vi "FOCUS_V42_H37.vi"(9 "X-pixels":sgl=256.0 min=2 step=2, 11 "Run":bool) -> (0 "Retrace pixels":sgl=32.0 min=2 step=2, 10 "Pixel Clock (Hz)":sgl=170000.0)   [LabVIEW 2010]
doc: "This Labview program is the user interface for a 2 photon imaging system. The acquisition and control hardware consists of 3 commercial boards from National Instruments. A PCI-6110E 4 channel 5MS/S 12 bit simultaneous-sampling analog input board is used for acquiring data. Two PCI-6711 analog output boards are used to generate the X and Y waveforms which drive the scanning mirrors. A number of custom VIs are used in addition to the standard VIs available with the base Labview development system and the Labview Vision module.\n\nDeveloped for the Kleinfeld Lab in the Physics Dept. at UCSD.\nRelease 1. May 2003."
uses:
  <vilib>/DAQmx/write.llb/DAQmx Write.vi
  <vilib>/DAQmx/create/channels.llb/DAQmx Create Virtual Channel.vi
  <vilib>/DAQmx/read.llb/DAQmx Read.vi
  <vilib>/DAQmx/configure/trigger.llb/DAQmx Trigger.vi
  <vilib>/DAQmx/configure/timing.llb/DAQmx Timing.vi
  <vilib>/Analysis/baseanly.llb/Real A x B.vi
  <vilib>/Analysis/NI_AALBase.lvlib
  <vilib>/Utility/inputDevices.llb/Close Input Device.vi
  FOCUS_V4.llb/GlobelFSCOPE.vi
  Program Files/National Instruments/LabVIEW 2010/resource/objmgr/daqmx.rc
  <vilib>/Analysis/1siggen.llb/Ramp Pattern by Samples.vi
panel:
  in  "Case Constant\n(See Context Help)":bool
  in  "Notebook Window":string="Date:\nType of experiment:\nStaining: "
  in  "Modes":T1(tab)=enum."Parameters"
  in  "Channel selector":u8(ring) items=["Green and Red", "Green and Blue", "Blue and Red", "Green and Red (and Blue)", "Green and Blue (and Red)", "Blue and Red (and Green)"]
  in  "Linescan mode":bool caption="Vertical\n\n\nHorizontal"
  in  "Focus":bool
  in  "OpenShutter":bool
  in  "Scale":u8(slide)=25 scale=1.0..254.0
  out "Hit Graph":u32[][](graph)
  in  "SlideHorizontal":u32(slide)
  in  "ImageSlide":u32(slide) scale=0.0..-1.0
  out "XY Graph 4":cluster{dbl[], dbl[]}(graph)
  out "XY Graph 3":cluster{dbl[], dbl[]}(graph)
  out "Histogram2":cluster{i32[], i32[]}(graph)
  out "Histogram1":cluster{i32[], i32[]}(graph)
  out "Image 4":u8[][](graph) caption="Image 2"
  out "Image 3":u8[][](graph)
  in  "Autosave":bool
  out "Save?":bool
  in  "Save? 2":bool
  in  "Open?":bool
  in  "Autoincrement Filename":bool
  in  "End experiment":bool
  out "Galvos":cluster{dbl[], dbl[]}(graph)
  out "Shutter open":bool
  out "Frame rate [Hz]":sgl=1.953125 format="%.2f"
  out "Ready?":bool=TRUE
  in  "stop 2":bool
  in  "Velocity":dbl(slide)=100.0 scale=200.0..1.0
  in  "Play Movie":bool
  out "Alexa value":sgl format="%#_6f"
  out "OGB value":sgl format="%#_6f"
  in  "Measurement cursor check box":bool
  in  "View line\ncheck box":bool
  in  "Parameters":T2(tab)
  in  "Test Run?":bool
  in  "Int Corr?":bool
  in  "Go back?":bool
  in  "Go further?":bool
  in  "Scale":sgl
  in  "Scanpattern":bool
  in  "Shift":sgl=-2.0000002 step=0.1
  in  "z frequency":dbl(slide) scale=0.0..20.0
  in  "Y-Scale":bool caption="Coarse\n\nFine"
  in  "Fiberscope\nMode":bool
  in  "Fiberscope":enum32{"Page 1"}(tab)
  out "Frame rate [Hz]":sgl=50000.0
  out "#":sgl=1.0
  out "#":sgl
  out "#":sgl
  in  "Number of Frames":sgl min=1
  in  "Averaging":sgl min=1
  in  "Number of Stacks":sgl min=1
  in  "Time interval [s]":sgl min=0
  in  "LS X/Y":bool=TRUE caption="LS X\n\n\n\nLS Y"
  in  "f min X":dbl
  in  "f max X":dbl=300.0
  in  "f min Y":dbl
  in  "f max Y":dbl=300.0
  in  "Zero 2":bool
  out "Focus":sgl min=1
  in  "Up 100":bool
  in  "Down 100":bool
  in  "Up 10":bool
  in  "Down 10":bool
  in  "Up 1":bool
  in  "Down 1":bool
  in  "Scan format FScope":u16(ring)=1 caption="Scan format" items=["user-defined ", "64 x 64", "128 x 128", "256 x 256", "512 x 512", "32 x 32"]
  in  "ScaleCluster":T3 {"Phase YX" scale=0.0..360.0; "Phase XY" scale=0.0..360.0; "Phase Y" scale=0.0..360.0; "Phase X" scale=0.0..360.0}
  in  "Y dim":sgl
  in  "X dim":sgl
  in  "scans to read":sgl
  in  "NewScanpattern":bool
  in  "Mode selectorFScope":u16(ring) items=["Focus mode", "Frame scan", "Straight line scan", "XY Graph"]
  in  "slope":i32(ring)=10280 items=["Rising"=10280, "Falling"=10171]
  in  "Level [V]":sgl=1.0
  in  "Type":bool caption="D                A"
  in  "Trigger?":bool
  out "#":sgl=1.0
  in  "Number of stacks":sgl=1.0 min=1 step=1
  in  "XScale":bool=TRUE caption="Fine              Coarse\n        X-Scale"
  in  "Scan format 2":u16(ring)=2 caption="Scan format" items=["10x objective", "20x objective", "40x objective", "60x objective"]
  in  "ImageSelector":bool caption="FreeLine\n\nStack"
  in  "line scan time (ms)":sgl=2.0 min=1 max=10 step=0.5
  in  "Time interval [s]":sgl
  in  "z-step (um)":sgl
  out "#":sgl=1000.0 min=2 step=2
  in  "Y-lines FreeLine":sgl min=2 step=2
  in  "Cusp Delay":sgl
  out "#":sgl=1.0
  in  "Number of frames":sgl=1.0 min=1 step=1
  in  "Amplitude Factor":sgl
  in  "phase shift [°]":sgl
  out "#":sgl=256.0
  in  "Y-lines":sgl=256.0 min=2 step=2
  out "#":sgl=1.0
  in  "Averaging":u16=1 min=1 step=1
  in  "Scan format":u16(ring)=3 items=["user-defined frame", "64 x 64, 2ms lines", "128 x 128, 2ms lines", "256 x 256, 2ms lines", "512 x 512, 2ms lines", "32 x 32, 1ms lines"]
  in  "FocusModeSelector":bool=TRUE
  in  "Mode selector":u16(ring) items=["Focus mode", "Frame scan", "Straight line scan", "FreeLine 2D", "Frame scan piezo", "FreeLine 3D"]
  in  "new FreeLine?":bool
  out "On?":bool
  in  "[µm] per pixel at zoom 1":sgl=0.39000058 min=0 step=0.01 format="%_2g"
  in  "Position piezo [µm]":sgl(slide)=200.0 caption="X amplitude" min=0 max=400 step=1 scale=0.0..400.0
  in  "Rotation z":sgl(slide)=90.0 caption="X amplitude" min=0 step=1 scale=0.0..90.0
  in  "scattering length [µm]":sgl=200.0 min=2 step=2
  in  "GetLast":bool
  in  "GetFirst":bool
  in  "IntensityAutomatic":bool caption="Automatic\n\nManual"
  in  "Reset":bool
  in  "Zoom 1":bool
  in  "Zero":bool
  in  "Offset Control":T4={"Up"=FALSE, "Left"=FALSE, "Down"=FALSE, "Right"=FALSE, "Zero"=FALSE, "Speed"=0.001, "UpLeft"=FALSE, "DownLeft"=FALSE, "UpRight"=FALSE, "DownRight"=FALSE} {"Speed" min=0.001 max=0.1 scale=0.0..0.1}
  out "IntDevUsed":bool
  in  "Intensity":sgl(slide)=0.1 caption="X amplitude" step=0.005 scale=0.0..1.0 scale format="%.2f"
  in  "Zoom":sgl(slide)=1.0 caption="X amplitude" min=0.28 step=0.01 scale=0.28..10.0 scale format="%.2f"
  in  "Rotation":sgl(knob) caption="rotation angle" min=0 max=360 scale=0.0..360.0
  out "colour table 2":u32[](array[colorbox])=[255, 0, 65793, 131586, 197379, 263172, 328965, 394758, 460551, 526344, 592137, 657930, 723723, 789516, 855309, 921102, 986895, 1052688, 1118481, 1184274, 1250067, 1315860, 1381653, 1447446, 1513239, 1579032, 1644825, 1710618, 1776411, 1842204, 1907997, 1973790, 2039583, 2105376, 2171169, 2236962, 2302755, 2368548, 2434341, 2500134, 2565927, 2631720, 2697513, 2763306, 2829099, 2894892, 2960685, 3026478, 3092271, 3158064, 3223857, 3289650, 3355443, 3421236, 3487029, 3552822, 3618615, 3684408, 3750201, 3815994, 3881787, 3947580, 4013373, 4079166, 4210752, 4276545, 4342338, 4408131, 4473924, 4539717, 4605510, 4671303, 4737096, 4802889, 4868682, 4934475, 5000268, 5066061, 5131854, 5197647, 5263440, 5329233, 5395026, 5460819, 5526612, 5592405, 5658198, 5723991, 5789784, 5855577, 5921370, 5987163, 6052956, 6118749, 6184542, 6250335, 6316128, 6381921, 6447714, 6513507, 6579300, 6645093, 6710886, 6776679, 6842472, 6908265, 6974058, 7039851, 7105644, 7171437, 7237230, 7303023, 7368816, 7434609, 7500402, 7566195, 7631988, 7697781, 7763574, 7829367, 7895160, 7960953, 8026746, 8092539, 8158332, 8224125, 8289918, 8355711, 8421504, 8487297, 8553090, 8618883, 8684676, 8750469, 8816262, 8882055, 8947848, 9013641, 9079434, 9145227, 9211020, 9276813, 9342606, 9408399, 9474192, 9539985, 9605778, 9671571, 9737364, 9803157, 9868950, 9934743, 10000536, 10066329, 10132122, 10197915, 10263708, 10329501, 10395294, 10461087, 10526880, 10592673, 10658466, 10724259, 10790052, 10855845, 10921638, 10987431, 11053224, 11119017, 11184810, 11250603, 11316396, 11382189, 11447982, 11513775, 11579568, 11645361, 11711154, 11776947, 11842740, 11908533, 11974326, 12040119, 12105912, 12171705, 12237498, 12303291, 12369084, 12434877, 12566463, 12632256, 12698049, 12763842, 12829635, 12895428, 12961221, 13027014, 13092807, 13158600, 13224393, 13290186, 13355979, 13421772, 13487565, 13553358, 13619151, 13684944, 13750737, 13816530, 13882323, 13948116, 14013909, 14079702, 14145495, 14211288, 14277081, 14342874, 14408667, 14474460, 14540253, 14606046, 14671839, 14737632, 14803425, 14869218, 14935011, 15000804, 15066597, 15132390, 15198183, 15263976, 15329769, 15395562, 15461355, 15527148, 15592941, 15658734, 15724527, 15790320, 15856113, 15921906, 15987699, 16053492, 16119285, 16185078, 16250871, 16316664, 16382457, 16448250, 16514043, 16579836, 16645629, 16711422, 16777215, 16711680]
  in  "Image Update [ms]":u32=50
  in  "VISA XPG-ADC":refnum<visa-resource-name>="COM4"
  in  "Different Integrator Setting":bool
  in  "Overlay Images":bool
  in  "Default colour table":bool
  in  "Different colour table":bool
  in  "2Ch\noverlay\nbutton":bool
  out "colour table":u32[](array[colorbox])=[255, 0, 65793, 131586, 197379, 263172, 328965, 394758, 460551, 526344, 592137, 657930, 723723, 789516, 855309, 921102, 986895, 1052688, 1118481, 1184274, 1250067, 1315860, 1381653, 1447446, 1513239, 1579032, 1644825, 1710618, 1776411, 1842204, 1907997, 1973790, 2039583, 2105376, 2171169, 2236962, 2302755, 2368548, 2434341, 2500134, 2565927, 2631720, 2697513, 2763306, 2829099, 2894892, 2960685, 3026478, 3092271, 3158064, 3223857, 3289650, 3355443, 3421236, 3487029, 3552822, 3618615, 3684408, 3750201, 3815994, 3881787, 3947580, 4013373, 4079166, 4210752, 4276545, 4342338, 4408131, 4473924, 4539717, 4605510, 4671303, 4737096, 4802889, 4868682, 4934475, 5000268, 5066061, 5131854, 5197647, 5263440, 5329233, 5395026, 5460819, 5526612, 5592405, 5658198, 5723991, 5789784, 5855577, 5921370, 5987163, 6052956, 6118749, 6184542, 6250335, 6316128, 6381921, 6447714, 6513507, 6579300, 6645093, 6710886, 6776679, 6842472, 6908265, 6974058, 7039851, 7105644, 7171437, 7237230, 7303023, 7368816, 7434609, 7500402, 7566195, 7631988, 7697781, 7763574, 7829367, 7895160, 7960953, 8026746, 8092539, 8158332, 8224125, 8289918, 8355711, 8421504, 8487297, 8553090, 8618883, 8684676, 8750469, 8816262, 8882055, 8947848, 9013641, 9079434, 9145227, 9211020, 9276813, 9342606, 9408399, 9474192, 9539985, 9605778, 9671571, 9737364, 9803157, 9868950, 9934743, 10000536, 10066329, 10132122, 10197915, 10263708, 10329501, 10395294, 10461087, 10526880, 10592673, 10658466, 10724259, 10790052, 10855845, 10921638, 10987431, 11053224, 11119017, 11184810, 11250603, 11316396, 11382189, 11447982, 11513775, 11579568, 11645361, 11711154, 11776947, 11842740, 11908533, 11974326, 12040119, 12105912, 12171705, 12237498, 12303291, 12369084, 12434877, 12566463, 12632256, 12698049, 12763842, 12829635, 12895428, 12961221, 13027014, 13092807, 13158600, 13224393, 13290186, 13355979, 13421772, 13487565, 13553358, 13619151, 13684944, 13750737, 13816530, 13882323, 13948116, 14013909, 14079702, 14145495, 14211288, 14277081, 14342874, 14408667, 14474460, 14540253, 14606046, 14671839, 14737632, 14803425, 14869218, 14935011, 15000804, 15066597, 15132390, 15198183, 15263976, 15329769, 15395562, 15461355, 15527148, 15592941, 15658734, 15724527, 15790320, 15856113, 15921906, 15987699, 16053492, 16119285, 16185078, 16250871, 16316664, 16382457, 16448250, 16514043, 16579836, 16645629, 16711422, 16777215, 16711680]
  out "Scan Backlock":u32
  in  "Scanblock Factor":sgl=4.0 min=0
  out "Scan Block Length":sgl=64.0
  out "Scan Parameters":T5={"X Pixels"=340.0, "Y Lines"=256.0, "Actual Line"=21760.0, "Zoom"=1.0, "X Offset"=0.0, "Y Offset"=0.0, " Rotation Angle (deg)"=0.0, " Lines to Generate"=21760.0} {"Rotation Angle (deg)" format="%.2f"; "Zoom" format="%.2f"; "Y Offset" format="%.2f"; "X Offset" format="%.2f"}
  out "NotebookFile":path
  out "Filename":string
  in  "BaseFilename":string
  in  "FilePath":path=path ""
  in  "Sutter Speed [um/s]":i32=700 min=1 step=1
  in  "MaiTai setting":bool
  in  "MaiTai setting Path":path=path "C:/Program Files/Spectra-Physics/Mai Tai rev D/Spectra-Physics Mai Tai.EXE"
  out "Shutter":refnum<k21>
  out "Intensity":refnum<k21>
  out "Data Input":refnum<k21>
  out "Scan Signals":refnum<k21>
  out "Position Signals":refnum<k21>
  out "Frame Clock":refnum<k21>
  out "Line Clock":refnum<k21>
  in  "VISA Sutter MP-285":refnum<visa-resource-name>="COM3"
  in  "AI Device":tag="PXI-6122"
  in  "AO/DIO Device":tag="PXI-6229"
  out "XY Graph 2":T6(graph)
  out "XY Graph 1":T6(graph)
  out "Image 1":u8[][](graph)
  out "Image 2":u8[][](graph)
  in  "F02":bool
  in  "F01":bool
  out "F01 2":sgl=nan
  in  "Background1":bool
  out "Background1 2":sgl=9.0
  in  "F0 1":bool
  in  "Reset2":bool
  in  "Background2":bool
  out "F02 2":sgl=nan
  in  "F0 2":bool
  out "Background2 2":sgl=9.0
  in  "Reset1":bool
  in  "Average2":i32=1 min=1
  in  "index (row)2":i32(slide) scale=0.0..99.0
  out "Profile2":cluster{dbl[], dbl[]}(graph)
  in  "Average1":i32=1 min=1
  in  "index (row)1":i32(slide) scale=0.0..99.0
  out "Profile1":cluster{dbl[], dbl[]}(graph)
  in  "Scangraph scaling":sgl=5.0 format="%_3g"
  out "CT1":bool
  out "CT2":bool
  in  "Sutter scale z":sgl=1.0 format="%_3g"
  in  "Sutter scale y":sgl=1.0 format="%_3g"
  in  "Sutter scale x":sgl=1.0 format="%_3g"
  out "Image3Arrayd":u8[][](array[numeric])
  out "frame scan finished?":bool
  out "Scan mode":u16(ring) items=["Retrace", "Back and forth"]
  in  "Scanner dead time":sgl=1300.0
  in  "Zoom 1 scan voltage":sgl=1.0
  in  "Stimulus Duration [s] 2":sgl=1.0 min=0
  in  "Interval [x Lines] 2":sgl=1.0 min=0 step=1
  in  "Stimulus Duration [s]":sgl=1.0 min=0
  in  "Interval [x Lines]":sgl=1.0 min=0 step=1
  in  "Stimulus":bool
  out "pixel dwell time [us] FreeLine":sgl format="%#_4f"
  out "LastPosition":sgl=256.0
  out "FirstPosition":sgl=-6406.57
  out "ParametersFScope":T7={"X frequeny [Hz]"=250, "Y frequency \n[Hz]"=128, "frequeny Trim"=0.0, "Samples/s"=50000, "Amplitude X"=1.0, "Amplitude Y"=1.0}
  out "Scanlength":sgl=64.0
  out "Pixel Clock (Hz) FScope":sgl format="%_2g"
  out "ScanLineFScope":sgl[][](array[numeric])=[[0.026666667, 0.10555588, 0.18413667, 0.2620946, 0.33912018, 0.4149288, 0.48917702, 0.5616217, 0.6319491, 0.69988036, 0.7651882, 0.8275282, 0.88674605, 0.9425593, 0.9947472, 1.043162, 1.087492, 1.127687, 1.163523, 1.1948596, 1.2216425, 1.2436236, 1.2608614, 1.2732126, 1.2806307, 1.2831601, 1.280641, 1.2732344, 1.2608918, 1.2436653, 1.2216938, 1.1949208, 1.1635948, 1.1277666, 1.0875816, 1.0432596, 0.9948533, 0.9426741, 0.8868671, 0.8276569, 0.7653226, 0.70002097, 0.6320957, 0.5617722, 0.48933217, 0.41508698, 0.33928153, 0.2622585, 0.18430196, 0.10572225, 0.026833316, -0.052056268, -0.13063815, -0.20859744, -0.28562555, -0.36143658, -0.43568876, -0.50813806, -0.57846946, -0.6464066, -0.71171933, -0.77406645, -0.833292, -0.8891114, -0.941308, -0.9897297, -1.0340693, -1.0742743, -1.110118, -1.1414653, -1.1682563, -1.1902486, -1.2074977, -1.2198576, -1.2272873, -1.2298253, -1.2273177, -1.2199228, -1.2075888, -1.1903737, -1.1684103, -1.1416483, -1.110333, -1.0745125, -1.0343375, -0.99002266, -0.9416256, -0.8894551, -0.83365417, -0.7744517, -0.71212274, -0.6468276, -0.57890815, -0.5085887, -0.43615317, -0.36191097, -0.28610873, -0.20908824, -0.13062674, -0.05199747], [-1.2831608, -1.2806358, -1.2732235, -1.2608767, -1.2436445, -1.2216686, -1.1948903, -1.163559, -1.1277268, -1.0875369, -1.0432112, -0.9948003, -0.94261676, -0.88680667, -0.8275926, -0.7652557, -0.69995075, -0.6320225, -0.56169707, -0.48925468, -0.41500804, -0.33920097, -0.26217666, -0.18421942, -0.105639175, -0.026750105, 0.052139297, 0.13072063, 0.20867924, 0.28570607, 0.3615159, 0.4357661, 0.5082131, 0.57854253, 0.6464767, 0.71178705, 0.7741306, 0.83335227, 0.88916856, 0.9413609, 0.9897791, 1.034114, 1.0743139, 1.1101538, 1.1414957, 1.1682826, 1.1902695, 1.2075129, 1.2198684, 1.2272923, 1.2298261, 1.2273127, 1.2199119, 1.2075737, 1.1903529, 1.1683854, 1.1416179, 1.1102973, 1.0744729, 1.034293, 0.98997456, 0.94157284, 0.889398, 0.833594, 0.7743877, 0.7120561, 0.6467577, 0.5788353, 0.50851387, 0.4360761, 0.3618324, 0.28602856, 0.20900682, 0.13105093, 0.052471776, -0.026417017, -0.10530679, -0.18388921, -0.2618492, -0.33887854, -0.4146908, -0.48894495, -0.56139654, -0.63172984, -0.69966996, -0.76498514, -0.82733583, -0.8865652, -0.94238764, -0.9945887, -1.0430137, -1.0873581, -1.127568, -1.1634157, -1.1947683, -1.2215633, -1.2435613, -1.260816, -1.2693994, -1.2762786]]
  in  "IntensityScaleMax":sgl=1.0 min=0 step=1
  in  "y offset":dbl step=0.005 format="%#_3g"
  in  "x offset":dbl step=0.005 format="%#_3g"
  in  "y scale":dbl=1.0 step=0.01
  in  "x scale":dbl=1.0 step=0.01
  out "ZInt3D":sgl[](array[numeric])
  out "ImageSlideMax":sgl
  out "Length1":dbl
  out "Index1":dbl
  out "Length2":dbl
  out "Index2":dbl
  out "x scan signals":dbl[](array[numeric]) format="%#_3g"
  out "y scan signals":dbl[](array[numeric]) format="%#_3g"
  out "Positions":sgl[](array[numeric])
  out "PointsCoordinates":i32[][](array[numeric])
  out "Image4Array":u8[][](array[numeric])
  out "Image3Array":u8[][](array[numeric])
  out "ScanSignals":dbl[][](array[numeric])
  out "Image2Array":u8[][](array[numeric])
  out "Image1Array":u8[][](array[numeric])
  out "Zsin3D":sgl[](array[numeric])
  out "ScanLineFreeLine":sgl[][](array[numeric])=[[0.026666667, 0.10555588, 0.18413667, 0.2620946, 0.33912018, 0.4149288, 0.48917702, 0.5616217, 0.6319491, 0.69988036, 0.7651882, 0.8275282, 0.88674605, 0.9425593, 0.9947472, 1.043162, 1.087492, 1.127687, 1.163523, 1.1948596, 1.2216425, 1.2436236, 1.2608614, 1.2732126, 1.2806307, 1.2831601, 1.280641, 1.2732344, 1.2608918, 1.2436653, 1.2216938, 1.1949208, 1.1635948, 1.1277666, 1.0875816, 1.0432596, 0.9948533, 0.9426741, 0.8868671, 0.8276569, 0.7653226, 0.70002097, 0.6320957, 0.5617722, 0.48933217, 0.41508698, 0.33928153, 0.2622585, 0.18430196, 0.10572225, 0.026833316, -0.052056268, -0.13063815, -0.20859744, -0.28562555, -0.36143658, -0.43568876, -0.50813806, -0.57846946, -0.6464066, -0.71171933, -0.77406645, -0.833292, -0.8891114, -0.941308, -0.9897297, -1.0340693, -1.0742743, -1.110118, -1.1414653, -1.1682563, -1.1902486, -1.2074977, -1.2198576, -1.2272873, -1.2298253, -1.2273177, -1.2199228, -1.2075888, -1.1903737, -1.1684103, -1.1416483, -1.110333, -1.0745125, -1.0343375, -0.99002266, -0.9416256, -0.8894551, -0.83365417, -0.7744517, -0.71212274, -0.6468276, -0.57890815, -0.5085887, -0.43615317, -0.36191097, -0.28610873, -0.20908824, -0.13062674, -0.05199747], [-1.2831608, -1.2806358, -1.2732235, -1.2608767, -1.2436445, -1.2216686, -1.1948903, -1.163559, -1.1277268, -1.0875369, -1.0432112, -0.9948003, -0.94261676, -0.88680667, -0.8275926, -0.7652557, -0.69995075, -0.6320225, -0.56169707, -0.48925468, -0.41500804, -0.33920097, -0.26217666, -0.18421942, -0.105639175, -0.026750105, 0.052139297, 0.13072063, 0.20867924, 0.28570607, 0.3615159, 0.4357661, 0.5082131, 0.57854253, 0.6464767, 0.71178705, 0.7741306, 0.83335227, 0.88916856, 0.9413609, 0.9897791, 1.034114, 1.0743139, 1.1101538, 1.1414957, 1.1682826, 1.1902695, 1.2075129, 1.2198684, 1.2272923, 1.2298261, 1.2273127, 1.2199119, 1.2075737, 1.1903529, 1.1683854, 1.1416179, 1.1102973, 1.0744729, 1.034293, 0.98997456, 0.94157284, 0.889398, 0.833594, 0.7743877, 0.7120561, 0.6467577, 0.5788353, 0.50851387, 0.4360761, 0.3618324, 0.28602856, 0.20900682, 0.13105093, 0.052471776, -0.026417017, -0.10530679, -0.18388921, -0.2618492, -0.33887854, -0.4146908, -0.48894495, -0.56139654, -0.63172984, -0.69966996, -0.76498514, -0.82733583, -0.8865652, -0.94238764, -0.9945887, -1.0430137, -1.0873581, -1.127568, -1.1634157, -1.1947683, -1.2215633, -1.2435613, -1.260816, -1.2693994, -1.2762786]]
  out "OriginalScanSignals":dbl[][](array[numeric])
  in  "reset?":dbl=125.0
  out "DataOffset":i32
  out "ScanLineLength":i32
  out "ZSinLength":i32
  out "DataLength":i32=131072
  out "Pixel Clock z (Hz) FreeLine":sgl=5.0 min=1 max=10 step=1 format="%_2g"
  out "Pixel Clock (Hz) FreeLine":sgl=5.0 min=1 max=10 step=1 format="%_2g"
  out "X-pixels FreeLine":sgl=100.0
  out "pixel dwell time [us]":sgl=5.882353 format="%#_4f"
  out "z-positionstop (um)":sgl=-6406.57
  out "x-positionstop (um)":sgl=-16582.2
  out "y-positionstop (um)":sgl=1941.2
  out "z-positionstart (um)":sgl=-4606.28
  out "x-positionstart (um)":sgl=-115939.0
  out "y-positionstart (um)":sgl=-86826.0
  out "Header":u8[](array[numeric])=[52, 48, 102, 105, 108, 101, 110, 97, 109, 101, 48, 48, 48, 48, 48, 48, 0, 0, 0, 0, 0, 0, 0, 0, 0, 0, 0, 0, 0, 0, 0, 0, 49, 53, 58, 48, 48, 0, 0, 0, 0, 0, 0, 0, 0, 0, 0, 0, 49, 50, 48, 52, 48, 54, 0, 0, 0, 0, 0, 0, 0, 0, 0, 0, 16, 52, 27, 230, 16, 52, 28, 150, 255, 158, 62, 86, 0, 0, 3, 0, 255, 2, 249, 201, 0, 29, 158, 208, 255, 2, 249, 201, 0, 29, 158, 208, 255, 158, 62, 86, 0, 0, 0, 0, 0, 0, 0, 0, 63, 128, 0, 0, 0, 0, 0, 0, 0, 0, 0, 0, 0, 0, 0, 0, 0, 0, 0, 0, 0, 0, 0, 0, 0, 0, 0, 0, 0, 0, 0, 0, 0, 0, 0, 0, 0, 0, 0, 0, 0, 0, 0, 0, 0, 0, 0, 0, 0, 0, 0, 0, 0, 0, 0, 0, 0, 0, 0, 0, 0, 0, 0, 0, 0, 0, 0, 0, 0, 0, 0, 0, 0, 0, 0, 0, 0, 0, 0, 0, 0, 0, 0, 0, 0, 0, 0, 0, 0, 0, 0, 0, 0, 0, 0, 0, 0, 0, 0, 0, 0, 0, 0, 0, 0, 0, 0, 0, 0, 0, 0, 0, 0, 0, 0, 0, 0, 0, 0, 0, 0, 0, 0, 0, 0, 0, 0, 0, 0, 0, 0, 0, 0, 0, 0, 0, 0, 0, 0, 0, 0, 0, 0, 0, 0, 0, 0, 0, 66, 128, 0, 0, 0, 0, 0, 0, 0, 0, 0, 0, 0, 0, 0, 0, 77, 34, 31, 232, 0, 0, 0, 0, 1, 0, 1, 0, 0, 0, 0, 0, 4, 0, 0, 0, 63, 128, 0, 0, 0, 0, 0, 0, 0, 0, 0, 0, 0, 0, 0, 0, 0, 1, 0, 0, 1, 0, 1, 0, 64, 0, 0, 0, 57, 69, 97, 7, 0, 0, 0, 0, 0, 0, 0, 0, 0, 0, 0, 0, 48, 48, 48, 48, 0, 0, 0, 0, 0, 0, 0, 0, 0, 0, 0, 0, 0, 0, 0, 0, 0, 0, 0, 0, 0, 0, 0, 0, 0, 0, 0, 0, 0, 0, 0, 0, 0, 0, 0, 0, 0, 0, 0, 0, 0, 0, 0, 0, 0, 0, 0, 0, 0, 0, 0, 0, 0, 0, 0, 0, 0, 0, 0, 0, 0, 0, 0, 0, 0, 0, 0, 0, 0, 0, 0, 0, 0, 0, 0, 0, 0, 0, 0, 0, 0, 0, 0, 0, 0, 0, 0, 0, 0, 0, 0, 0, 0, 0, 0, 0, 0, 0, 0, 0, 0, 0, 0, 0, 0, 0, 0, 0, 0, 0, 0, 0, 0, 0, 0, 0, 0, 0, 0, 0, 0, 0, 0, 0, 0, 0, 0, 0, 0, 0, 0, 0, 0, 0, 0, 0, 0, 0, 0, 0, 0, 0, 0, 0, 0, 0, 0, 0, 0, 0, 0, 0, 0, 0, 0, 0, 0, 0, 0, 0, 0, 0, 0, 0, 0, 0, 0, 0, 0, 0, 0, 0, 2, 188, 2, 187, 0, 0, 0, 0, 0, 0, 0, 0, 0, 0, 0, 0, 63, 128, 0, 0, 63, 128, 0, 0, 0, 0, 0, 0, 0, 0, 0, 0, 0, 0, 0, 0, 0, 0, 0, 0, 0, 0, 0, 0, 0, 0, 0, 0, 0, 0, 0, 0, 0, 0, 0, 0, 0, 0, 0, 0, 0, 0, 0, 0, 66, 200, 0, 0, 0, 0, 0, 0, 64, 160, 0, 0, 0, 0, 0, 0, 0, 0, 0, 0, 64, 160, 0, 0, 0, 0, 0, 0, 0, 0, 0, 0, 0, 0, 0, 0, 0, 0, 0, 0, 0, 0, 0, 1, 0, 0, 0, 0, 0, 0, 0, 0, 0, 0, 0, 0, 0, 0, 0, 0, 0, 0, 0, 0, 0, 0, 0, 0, 0, 0, 0, 0, 0, 0, 0, 0, 0, 0, 0, 0, 0, 0, 0, 0, 0, 0, 0, 0, 0, 0, 0, 0, 0, 0, 0, 0, 0, 0, 0, 0, 0, 0, 0, 0, 0, 0, 0, 0, 0, 0, 0, 0, 0, 0, 0, 0, 0, 0, 0, 0, 0, 0, 0, 0, 0, 0, 0, 0, 0, 0, 0, 0, 0, 0, 0, 0, 0, 0, 0, 0, 0, 0, 0, 0, 0, 0, 0, 0, 0, 0, 0, 0, 0, 0, 0, 0, 0, 0, 0, 0, 0, 0, 0, 0, 0, 0, 0, 0, 0, 0, 0, 0, 0, 0, 0, 0, 0, 0, 0, 0, 0, 2, 0, 0, 0, 0, 0, 0, 0, 0, 0, 0]
  out "Program Version":u16=13362
  out "stop":u32=271850646
  out "start":u32=271850470
  out "pixels in frame + yretrace":sgl=65536.0
  out "pixels in frame":sgl=65536.0
  out "total pixels in frame":sgl=87040.0
  out "Time":string="10:33"
  out "Date":string="011607"
  out "pixelstoµm":sgl=100.0 min=2 step=2
  in  "x-step (um)":sgl
  in  "y-step (um)":sgl
  out "frame/line indicator":u16(ring) items=["focus", "frame", "line", "user-defined line", "3D user-defined line"]
  out "total y pixels":sgl=256.0
  out "total x pixels":sgl=340.0
  in  "y jog":sgl=0.432538
  in  "x jog":sgl=-0.66191
  out "Scan Cut-Off (either end)":sgl=26.0 min=0 max=4095 step=1
  out "Program Version":string="4.2"
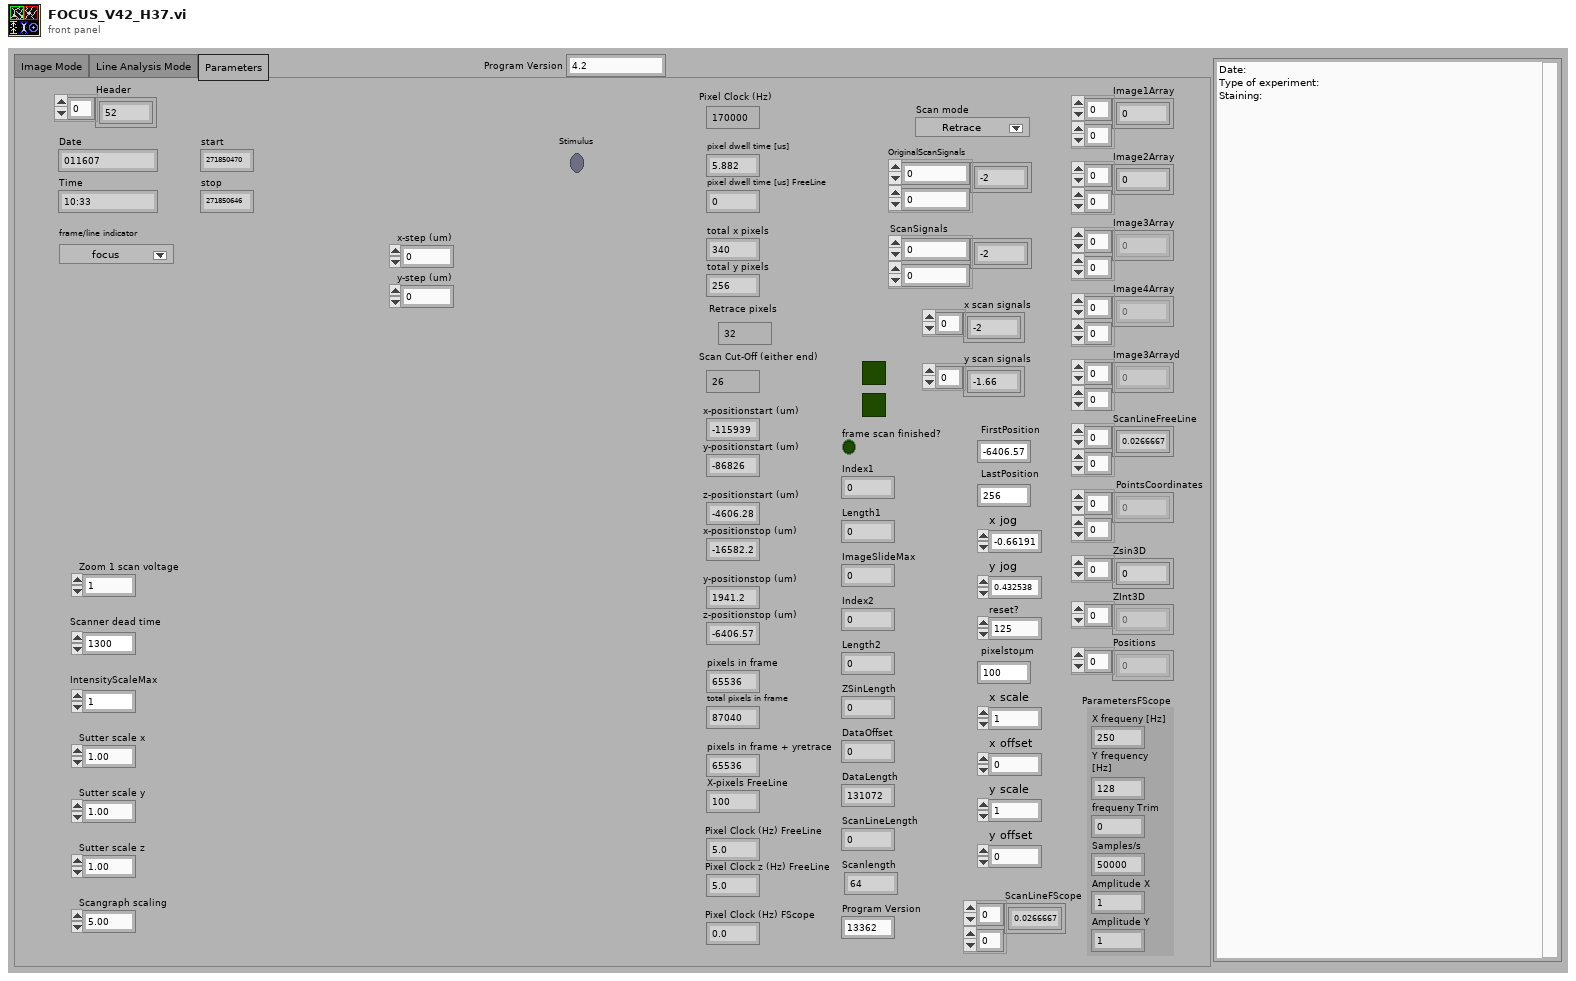
[diagram p1: front panel]
types:
  T1 = enum32{"Image Mode", "Line Analysis Mode", "Parameters"}
  T2 = enum32{"Scan Mode", "Offset Rotation", "Image Manipulation", "Scan Parameters", "File Path Parameters", "Device Parameters"}
  T3 = cluster{"Phase X":dbl, "Phase Y":dbl, "Amplitude YX":dbl, "Amplitude XY":dbl, "Phase XY":dbl, "Phase YX":dbl}
  T4 = cluster{"Up":bool, "Left":bool, "Down":bool, "Right":bool, "Zero":bool, "Speed":sgl, "UpLeft":bool, "DownLeft":bool, "UpRight":bool, "DownRight":bool}
  T5 = cluster{"X Pixels":sgl, "Y Lines":sgl, "Actual Line":sgl, "Zoom":sgl, "X Offset":sgl, "Y Offset":sgl, " Rotation Angle (deg)":sgl, " Lines to Generate":sgl}
  T6 = cluster{"x voltages":dbl[], "y voltages":dbl[]}[]
  T7 = cluster{"X frequeny [Hz]":i32, "Y frequency \n[Hz]":i32, "frequeny Trim":dbl, "Samples/s":i32, "Amplitude X":dbl, "Amplitude Y":dbl}
  T8 = enum16{"open", "open or create", "create or replace", "create", "open (read only)"}
  T9 = cluster{"X frequeny [Hz]":bool, "Y frequency \n[Hz]":bool, "frequeny Trim":bool, "Samples/s":bool, "Amplitude X":bool, "Amplitude Y":bool}
  T10 = enum32{"existing file", "new file", "new or existing file", "existing dir", "new dir", "new or existing dir", "existing file (use LLBs)", "new file (use LLBs)", "new or existing file (use LLBs)", "new or existing file or directory (use LLBs)"}
  T11 = cluster{"X frequeny [Hz]":i32, "X frequeny [Hz]":i32, "frequeny Trim":dbl, "Samples/s":i32, "Amplitude X":dbl, "Amplitude X":dbl}
  T12 = enum16{"deny read/write", "deny write-only", "deny none"}
  T13 = cluster{"frame/line indicator":u16, "X-pixels":sgl, "Y-lines":sgl, "line scan time (ms)":sgl, "Zoom 1 scan voltage":sgl, "Scanblock Factor":sgl, "Scanpattern":bool}
  T14 = cluster{"Scan mode":u16, "Pixel Clock (Hz)":sgl, "pixel dwell time [us]":sgl, "Frame rate (Hz)":sgl, "total x pixels":sgl, "total y lines":sgl, "Retrace pixels (tdown)":sgl, "Scan Cut-Off (either end)":sgl, "pixels in frame":sgl, "pixels in frame + yretrace":sgl, "Scanblock length":sgl, "total pixels in frame":sgl, "Z-scan mode":u16}
  T15 = typedef "NI_Matrix.lvlib/RealMatrix.ctl" = dbl[][]
  T16 = cluster{" PointsCoordinates":i32[], " PointsCoordinates":i32[]}
  T17 = cluster{"Trigger?":bool, "Type":bool, "Level [V]":sgl, "slope":i32}
  T18 = cluster{"Output: VISA session OUT":refnum<visa-resource-name>, "Error cluster":errorcluster}
  T19 = cluster{"BaseFilename":string, "FilePath":path, "Autoincrement Filename":bool, bool}
  T20 = cluster{"ScaleCluster":cluster{"Phase X":dbl, "Phase Y":dbl, "Amplitude YX":dbl, "Amplitude XY":dbl, "Phase XY":dbl, "Phase YX":dbl}, "scans to read":sgl}
  T21 = cluster{"Program Version":u16, "name":string, "Time":string, "Date":string, "start":u32, "stop":u32, "IntDevUsed":bool, "Intensity":sgl, "Scan Block Length":sgl, "Pixel Clock (Hz)":sgl, "X-pixels":sgl, "Y-lines":sgl, "Number of frames":sgl, "Averaging":u16, "line scan time (ms)":sgl, "Retrace pixels":sgl, "z-step (um)":sgl, "x-step (um)":sgl, "y-step (um)":sgl, dbl, dbl, "x jog":sgl, "y jog":sgl, "Rotation":sgl, "Zoom":sgl, "Number of stacks":sgl, "Time interval [s]":sgl, cluster{"z-positionstart (um)":sgl, "x-positionstart (um)":sgl, "y-positionstart (um)":sgl, "x-positionstop (um)":sgl, "y-positionstop (um)":sgl, "z-positionstop (um)":sgl, "X-pixels FreeLine":sgl, "Y-lines FreeLine":sgl, "Pixel Clock (Hz) FreeLine":sgl, "Amplitude Factor":sgl, "Pixel Clock z (Hz) FreeLine":sgl, "phase shift [°]":sgl, "Mode selector":u16, "Cusp Delay":sgl, "Fiberscope\nMode":bool, "Pixel Clock (Hz) FScope":sgl, "scans to read":sgl, "LS X/Y":bool, "DataOffset":i32, "DataLength":i32, "ScanLineLength":i32, "ZSinLength":i32}}
  T22 = cluster{"z-positionstart (um)":sgl, "x-positionstart (um)":sgl, "y-positionstart (um)":sgl, "x-positionstop (um)":sgl, "y-positionstop (um)":sgl, "z-positionstop (um)":sgl, "X-pixels FreeLine":sgl, "Y-lines FreeLine":sgl, "Pixel Clock (Hz) FreeLine":sgl, "Amplitude Factor":sgl, "Pixel Clock z (Hz) FreeLine":sgl, "phase shift [°]":sgl, "Mode selector":u16, "Cusp Delay":sgl, "Fiberscope\nMode":bool, "Pixel Clock (Hz) FScope":sgl, "scans to read":sgl, "LS X/Y":bool, "DataOffset":i32, "DataLength":i32, "ScanLineLength":i32, "ZSinLength":i32}
  T23 = cluster{"ScanLineUDL":sgl[], "ScanLineUDL":sgl[]}
  T24 = cluster{"ScanLineUDL":sgl[], "ScanLineUDL":sgl[]}[]
  T25 = typedef "LVRectTypeDef.ctl" = cluster{"left":i16, "top":i16, "right":i16, "bottom":i16}
  T26 = cluster{sgl, sgl, sgl, "Zoom":sgl, "x jog":sgl, "y jog":sgl, sgl, sgl, "Rotation z":sgl, sgl, " [µm] per pixel at zoom 1":sgl, "Intensity":sgl, "scattering length [µm]":sgl}
  T27 = cluster{"X Pixels":sgl, "Y Lines":sgl, "Actual Line":sgl, "Zoom":sgl, "X Offset":sgl, "Y Offset":sgl, " Rotation Angle (deg)":sgl, " Lines to Generate":sgl, "Rotation z":sgl, "Position piezo":sgl, "z scaling":sgl, "Intensity":sgl, "Scattering length (um)":sgl}
  T28 = cluster{"Horizontal":i32, "Vertical":i32, "Scrolling":i32}
  T29 = cluster{"button 1":bool, "button 2":bool, "button 3":bool, "button 4":bool}
  T30 = cluster{"X Pixels":sgl, "Y Lines":sgl, "Actual Line":sgl, "Zoom":sgl, sgl, sgl, " Rotation Angle (deg)":sgl, " Lines to Generate":sgl, "Rotation z":sgl, "Position piezo":sgl, "z scaling":sgl, "Intensity":sgl, "Scattering length (um)":sgl}
  T31 = cluster{"scan signals":dbl[], "scan signals":dbl[]}
  T32 = cluster{sgl, sgl, sgl, "Zoom":sgl, "x jog":sgl, "y jog":sgl, sgl, sgl}
  T33 = cluster{"x offset":dbl, "x offset":dbl, "x offset":dbl, "x offset":dbl}
  T34 = cluster{"x offset":dbl, "x scale":dbl, "y offset":dbl, "y scale":dbl}
  T35 = cluster{"BaseFilename":string, "FilePath":path, "Autoincrement\nFilename":bool, bool}
  T36 = cluster{"Output: VISA session OUT":refnum<visa-resource-name>, "error out":errorcluster}
diagram:
  w26 = 4 ("length")
  w28 = 4 ("length")
  w33 = 1 ("index")
  w87 = "4.2" ("String")
  w37 = u32[] [255, 0, 65793, 131586, 197379, 263172, 328965, 394758, 460551, 526344, 592137, 657930, 723723, 789516, 855309, 921102, 986895, 1052688, 1118481, 1184274, 1250067, 1315860, 1381653, 1447446, 1513239, 1579032, 1644825, 1710618, 1776411, 1842204, 1907997, 1973790, 2039583, 2105376, 2171169, 2236962, 2302755, 2368548, 2434341, 2500134, 2565927, 2631720, 2697513, 2763306, 2829099, 2894892, 2960685, 3026478, 3092271, 3158064, 3223857, 3289650, 3355443, 3421236, 3487029, 3552822, 3618615, 3684408, 3750201, 3815994, 3881787, 3947580, 4013373, 4079166, 4210752, 4276545, 4342338, 4408131, 4473924, 4539717, 4605510, 4671303, 4737096, 4802889, 4868682, 4934475, 5000268, 5066061, 5131854, 5197647, 5263440, 5329233, 5395026, 5460819, 5526612, 5592405, 5658198, 5723991, 5789784, 5855577, 5921370, 5987163, 6052956, 6118749, 6184542, 6250335, 6316128, 6381921, 6447714, 6513507, 6579300, 6645093, 6710886, 6776679, 6842472, 6908265, 6974058, 7039851, 7105644, 7171437, 7237230, 7303023, 7368816, 7434609, 7500402, 7566195, 7631988, 7697781, 7763574, 7829367, 7895160, 7960953, 8026746, 8092539, 8158332, 8224125, 8289918, 8355711, 8421504, 8487297, 8553090, 8618883, 8684676, 8750469, 8816262, 8882055, 8947848, 9013641, 9079434, 9145227, 9211020, 9276813, 9342606, 9408399, 9474192, 9539985, 9605778, 9671571, 9737364, 9803157, 9868950, 9934743, 10000536, 10066329, 10132122, 10197915, 10263708, 10329501, 10395294, 10461087, 10526880, 10592673, 10658466, 10724259, 10790052, 10855845, 10921638, 10987431, 11053224, 11119017, 11184810, 11250603, 11316396, 11382189, 11447982, 11513775, 11579568, 11645361, 11711154, 11776947, 11842740, 11908533, 11974326, 12040119, 12105912, 12171705, 12237498, 12303291, 12369084, 12434877, 12566463, 12632256, 12698049, 12763842, 12829635, 12895428, 12961221, 13027014, 13092807, 13158600, 13224393, 13290186, 13355979, 13421772, 13487565, 13553358, 13619151, 13684944, 13750737, 13816530, 13882323, 13948116, 14013909, 14079702, 14145495, 14211288, 14277081, 14342874, 14408667, 14474460, 14540253, 14606046, 14671839, 14737632, 14803425, 14869218, 14935011, 15000804, 15066597, 15132390, 15198183, 15263976, 15329769, 15395562, 15461355, 15527148, 15592941, 15658734, 15724527, 15790320, 15856113, 15921906, 15987699, 16053492, 16119285, 16185078, 16250871, 16316664, 16382457, 16448250, 16514043, 16579836, 16645629, 16711422, 16777215, 16711680] ("Array")
  w100 = TRUE
  w101 = FALSE
  # "PFI lines:\nPFI 1   - shutter\nPFI 2   - 10MHz Ref Clock (PXI_Trig2)\nPFI 5   - Pixel Clock (PXI_Trig5)\nPFI 6   - Trigger Input\nPFI 7   - AO Start Trigger\nPFI 12 - line clock (CTR 0 OUT)\nPFI 13 - frame clock (CTR 1 OUT)\nPFI 14 - Motor Command\nPFI 15 - Motor Up / Down"
  n1 = property on="Property Node" class="VI"() -> ("VI Path"=w74:path)  [unwired: 2 in, 2 out]
  n2 = Strip Path(path=w74) -> (stripped path=w43:path)  [unwired: 1 out]
  n3 = Strip Path(path=w43) -> ()  [unwired: 2 out]
  n4 = local read "ParametersFScope"() -> (w22:T7)
  n5 = Path to Array of Strings(0:"FilePath") -> (2:w81:string[])  [unwired: 1 out]
  n6 = Build Path(base path=w43, name or relative path="FOCUS.cfg") -> (appended path=w62:path)
  n7 = String Length(string="BaseFilename") -> (length=w79:i32)
  n8 = Array Size(array=w81) -> (size(s)=w80:i32)
  n9 = Equal To 0?(x=w79) -> (x = 0?=w77:bool)
  n10 = Equal To 0?(x=w80) -> (x = 0?=w78:bool)
  n11 = local read "ScanLineFreeLine"() -> (w92:sgl[][])
  n12 = local read "ScanLineFScope"() -> (w23:sgl[][])
  n13 = Or(x=w78, y=w77) -> (x .or. y?=w76:bool)
  n14 = Equal?(x=w22, y=0.0 ("frequeny Trim")) -> (x = y?=w20:T9)
  n15 = call <vilib>:"Open_Create_Replace File.vi"("function (open:0)"=T8."open", "file path"=w62) -> ("error out"=w60:errorcluster, "file size (bytes)"=w59:i32, "refnum"=w61:refnum<file>)  [unwired: 6 in, 1 out]
  n16 = case shown="True" w76 {
    tunnel: [w102 w104] -> w7
    tunnel: "FilePath" -> [w102 _]
    frame False {
    }
    frame True {
      (unwired) T10."new or existing file" ("select mode (2)")
      n17 = Format Date/Time String(time format string (%c)="%m%d%y") -> (date/time string=w108:string)  [unwired: 2 in]
      n18 = Concatenate Strings("*_", w108, ".fcs") -> (w106:string)
      n19 = File Dialog(9:w106) -> (0:w103:errorcluster, 3:w107:path)  [unwired: 6 in, 2 out]
      n20 = Unbundle(w103) -> ()  [unwired: 3 out]
      n21 = Strip Path(path=w107) -> (stripped path=w104:path, name=w105:string)
      n22 = local write "BaseFilename"(w105) -> ()
      n23 = local write "FilePath"(w104) -> ()
    }
  }
  n24 = List Folder(path=w7, pattern="*.txt" ("string")) -> (filenames=w10:string[])  [unwired: 2 in, 3 out]
  n25 = Array Size(array=w10) -> (size(s)=w13:i32)
  n26 = Equal To 0?(x=w13) -> (x = 0?=w12:bool)
  n27 = case shown="False" w12 {
    tunnel: w10 -> [w130 _]
    tunnel: w7 -> [w115 _]
    tunnel: [w113 w139] -> w8
    frame False {
      n28 = for {
        tunnel: w130 -> [w138] mode=indexing
        tunnel: [w134] -> w129 mode=indexing
        n29 = Reverse String(1:w138) -> (0:w137:string)
        n30 = String Subset(string=w137, offset (0)=4, length (rest)=3 ("length (rest)")) -> (substring=w132:string)
        n31 = Reverse String(1:w132) -> (0:w131:string)
        n32 = Decimal String To Number(string=w131, default (0L)=u32 0 ("default (0 I32)")) -> (number=w134:u32)  [unwired: 1 in, 1 out]
      }
      n33 = Format Date/Time String(time format string (%c)="%m%d%y") -> (date/time string=w119:string)  [unwired: 2 in]
      n34 = Array Max & Min(array=w129) -> (max value=w128:u32)  [unwired: 3 out]
      n35 = Increment(x=w128) -> (x+1=w127:u32)
      n36 = Format Into String(w127) -> (resulting string=w122:string)  [unwired: 3 in, 1 out]
      n37 = String Length(string=w122) -> (length=w126:i32)
      n38 = Subtract(x=3, y=w126) -> (x-y=w123:i32)
      n39 = String Subset(string="000", length (rest)=w123) -> (substring=w116:string)  [unwired: 1 in]
      n40 = Concatenate Strings(w116, w122) -> (w114:string)
      n41 = Concatenate Strings("FOCUS_NOTEBOOK_" ("string"), w119, "_" ("string"), w114, ".txt" ("string")) -> (w117:string)
      n42 = Build Path(base path=w115, name or relative path=w117) -> (appended path=w113:path)
    }
    frame True {
      n43 = Format Date/Time String(time format string (%c)="%m%d%y") -> (date/time string=w143:string)  [unwired: 2 in]
      n44 = Concatenate Strings("FOCUS_NOTEBOOK_" ("string"), w143, "_000" ("string"), ".txt" ("string")) -> (w146:string)
      n45 = local read "FilePath"() -> (w141:path)
      n46 = Build Path(base path=w141, name or relative path=w146) -> (appended path=w139:path)
    }
  }
  "NotebookFile" <- w8
  n47 = Unbundle(w20) -> ("X frequeny [Hz]"=w19:bool, "Y frequency \n[Hz]"=w18:bool, "Amplitude X"=w17:bool, "Amplitude Y"=w16:bool)  [unwired: 2 out]
  n48 = Read from Binary File(5:u8 0 ("x 2"), 8:w60, 10:w59, 11:w61) -> (0:w72:errorcluster, 2:w35:u8[], 3:w71:refnum<file>)  [unwired: 2 in, 1 out]
  n49 = Array Size(array=w92) -> (size(s)=w95:i32[])
  n50 = Compound Arithmetic op=AND(w19, w18, w17, w16) -> (w15:bool)
  n51 = Array Size(array=w23) -> (size(s)=w40:i32[])
  n52 = Close File(refnum=w71, error in=w72) -> (error out=w70:errorcluster)  [unwired: 1 out]
  n53 = Multiply Array Elements(1:w95) -> (0:w94:i32)
  n54 = case shown="True" w15 {
    frame False {
    }
    frame True {
      w148 = 1.0 ("Amplitude X")
      n55 = Bundle("X frequeny [Hz]"=250, "X frequeny [Hz]"=128, "frequeny Trim"=0.0, "Samples/s"=50000, "Amplitude X"=w148, "Amplitude X"=w148) -> (w147:T11)  [unwired: 1 in]
      n56 = local write "ParametersFScope"(w147) -> ()
    }
  }
  n57 = Multiply Array Elements(1:w40) -> (0:w39:i32)
  n58 = Index Array(array=w35, index=0) -> (element=w34:u8)
  n59 = Add(x=w34, y=w33) -> (x+y=w32:i32)
  n60 = Index Array(array=w35, index=w32) -> (element=w30:u8)
  n61 = Array Subset(array=w35, index=w33, length=w34) -> (w68:u8[])
  n62 = property on="Notebook Window" class="Str"("Text.Text"="Date:\nType of experiment:\nStaining: ") -> ()  [unwired: 2 in, 2 out]
  n63 = String Subset(string=w87, offset (0)=0, length (rest)=1 ("length (rest)")) -> (substring=w86:string)
  n64 = String Subset(string=w87, offset (0)=2, length (rest)=1 ("length (rest)")) -> (substring=w85:string)
  n65 = Equal To 0?(x=w94) -> (x = 0?=w93:bool)
  n66 = Equal To 0?(x=w39) -> (x = 0?=w38:bool)
  n67 = local write "LS X/Y"(TRUE ("LS X/Y")) -> ()
  n68 = Increment(x=w32) -> (x+1=w31:i32)
  n69 = Add(x=w31, y=w30) -> (x+y=w29:i32)
  n70 = Array Subset(array=w35, index=w31, length=w30) -> (w65:u8[])
  n71 = Array Subset(array=w35, index=w29, length=w28) -> (w56:u8[])
  n72 = Add(x=w29, y=w28) -> (x+y=w27:i32)
  n73 = Array Subset(array=w35, index=w27, length=w26) -> (w52:u8[])
  n74 = Add(x=w27, y=w26) -> (x+y=w25:i32)
  n75 = Index Array(array=w35, index=w25) -> (element=w46:u8)
  n76 = call <vilib>:"Simple Error Handler.vi"("error in (no error)"=w70) -> ()  [unwired: 4 in, 5 out]
  n77 = Type Cast(type="" ("name or relative path"), x=w52) -> (*(type *) &x=w50:string)
  n78 = Type Cast(type="" ("name or relative path"), x=w56) -> (*(type *) &x=w54:string)
  n79 = Increment(x=w25) -> (x+1=w24:i32)
  n80 = Array Subset(array=w35, index=w24, length=w46) -> (w48:u8[])
  n81 = property on="Image 1" class="IntGraph (strict)"("Color Table"=w37) -> ()  [unwired: 2 in, 2 out]
  n82 = Type Cast(type=tag "" ("6229 Device 2"), x=w68) -> (*(type *) &x=w67:tag)
  n83 = case shown="True" w93 {
    frame False {
    }
    frame True {
      w158 = sgl 5.0 ("Pixel Clock (Hz) udl")
      n84 = local write "Pixel Clock (Hz) FreeLine"(w158) -> ()
      n85 = local write "Pixel Clock z (Hz) FreeLine"(w158) -> ()
      n86 = local write "X-pixels FreeLine"(sgl 100.0 ("number of pixels udl")) -> ()
      n87 = local write "ScanLineFreeLine"(sgl[][] [[0.026666667, 0.10555588, 0.18413667, 0.2620946, 0.33912018, 0.4149288, 0.48917702, 0.5616217, 0.6319491, 0.69988036, 0.7651882, 0.8275282, 0.88674605, 0.9425593, 0.9947472, 1.043162, 1.087492, 1.127687, 1.163523, 1.1948596, 1.2216425, 1.2436236, 1.2608614, 1.2732126, 1.2806307, 1.2831601, 1.280641, 1.2732344, 1.2608918, 1.2436653, 1.2216938, 1.1949208, 1.1635948, 1.1277666, 1.0875816, 1.0432596, 0.9948533, 0.9426741, 0.8868671, 0.8276569, 0.7653226, 0.70002097, 0.6320957, 0.5617722, 0.48933217, 0.41508698, 0.33928153, 0.2622585, 0.18430196, 0.10572225, 0.026833316, -0.052056268, -0.13063815, -0.20859744, -0.28562555, -0.36143658, -0.43568876, -0.50813806, -0.57846946, -0.6464066, -0.71171933, -0.77406645, -0.833292, -0.8891114, -0.941308, -0.9897297, -1.0340693, -1.0742743, -1.110118, -1.1414653, -1.1682563, -1.1902486, -1.2074977, -1.2198576, -1.2272873, -1.2298253, -1.2273177, -1.2199228, -1.2075888, -1.1903737, -1.1684103, -1.1416483, -1.110333, -1.0745125, -1.0343375, -0.99002266, -0.9416256, -0.8894551, -0.83365417, -0.7744517, -0.71212274, -0.6468276, -0.57890815, -0.5085887, -0.43615317, -0.36191097, -0.28610873, -0.20908824, -0.13062674, -0.05199747], [-1.2831608, -1.2806358, -1.2732235, -1.2608767, -1.2436445, -1.2216686, -1.1948903, -1.163559, -1.1277268, -1.0875369, -1.0432112, -0.9948003, -0.94261676, -0.88680667, -0.8275926, -0.7652557, -0.69995075, -0.6320225, -0.56169707, -0.48925468, -0.41500804, -0.33920097, -0.26217666, -0.18421942, -0.105639175, -0.026750105, 0.052139297, 0.13072063, 0.20867924, 0.28570607, 0.3615159, 0.4357661, 0.5082131, 0.57854253, 0.6464767, 0.71178705, 0.7741306, 0.83335227, 0.88916856, 0.9413609, 0.9897791, 1.034114, 1.0743139, 1.1101538, 1.1414957, 1.1682826, 1.1902695, 1.2075129, 1.2198684, 1.2272923, 1.2298261, 1.2273127, 1.2199119, 1.2075737, 1.1903529, 1.1683854, 1.1416179, 1.1102973, 1.0744729, 1.034293, 0.98997456, 0.94157284, 0.889398, 0.833594, 0.7743877, 0.7120561, 0.6467577, 0.5788353, 0.50851387, 0.4360761, 0.3618324, 0.28602856, 0.20900682, 0.13105093, 0.052471776, -0.026417017, -0.10530679, -0.18388921, -0.2618492, -0.33887854, -0.4146908, -0.48894495, -0.56139654, -0.63172984, -0.69966996, -0.76498514, -0.82733583, -0.8865652, -0.94238764, -0.9945887, -1.0430137, -1.0873581, -1.127568, -1.1634157, -1.1947683, -1.2215633, -1.2435613, -1.260816, -1.2693994, -1.2762786]] ("transposed array")) -> ()
      n88 = Initialize Array(sgl 0.0 ("element"), 10 ("dimension size")) -> (w156:sgl[])
      n89 = local write "Zsin3D"(w156) -> ()
    }
  }
  n90 = local write "Run"(w101) -> ()
  n91 = Concatenate Strings(w86, w85) -> (w84:string)
  n92 = Negate(x="Scangraph scaling") -> (-x=w2:sgl)
  n93 = Negate(x="Scangraph scaling") -> (-x=w3:sgl)
  n94 = case shown="True" w38 {
    frame False {
    }
    frame True {
